vi "Read_Joint_States.vi"(0 "error in":errorcluster, 2 "Units (deg)":enum16{"Radians", "Degrees"}(ring)=enum."Degrees", 3 "node":string) -> (1 "error out":errorcluster, 4 "Joint States":T1(array[cluster]))   [LabVIEW 2015]
doc: "Read all the current joint states (names, positions, velocity, and efforts)"
uses:
  ROS/Code/Console/Servers/ServerSubs/TopicDef.ctl
  ROS/Code/SubVIs/_ROSDirection.ctl
panel:
  out "Reply":string
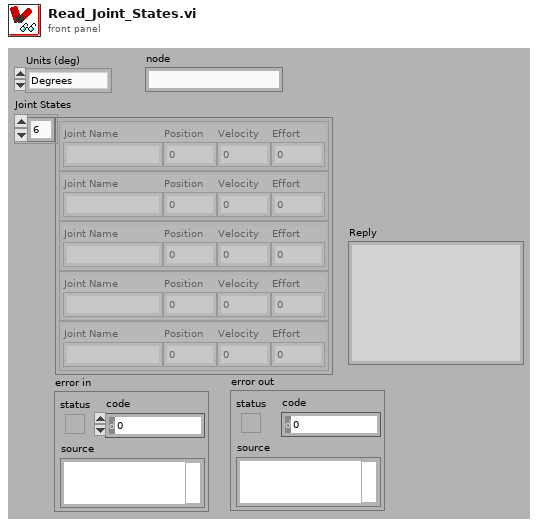
[diagram p1: front panel]
types:
  T1 = cluster{"Joint Name":string, "Position":dbl, "Velocity":dbl, "Effort":dbl}[]
  T2 = typedef "TopicDef.ctl" = cluster{"Topic":string, "Type":string, "Action":T3, "Update (ms)":u16, "queue size":u16}
  T3 = typedef "_ROSDirection.ctl" = enum16{"Node", "Publisher", "Subscriber", "ServiceClient", "ServiceProvider"}
  T4 = typedef "_ROSControl.ctl" = cluster{"topic port":u16, "Node":string, "topic":string, "type":string, "node port":u16, "error ":errorcluster, "Direction":T3, "Update (ms)":u16, "FIFO size":u16}
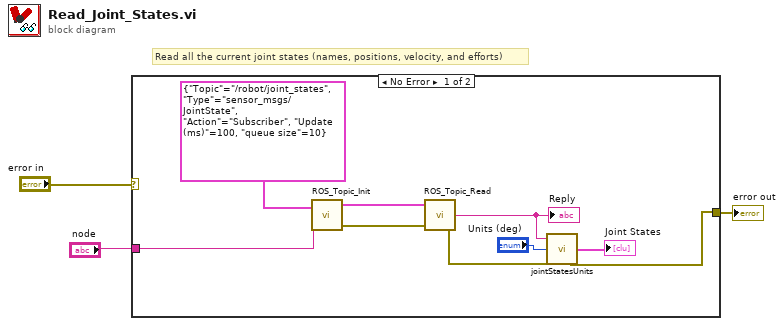
[diagram p0: block diagram]
diagram:
  # "Read all the current joint states (names, positions, velocity, and efforts)"
  n1 = case shown="No Error" "error in" {
    selector: "error in" -> [_ w13]
    tunnel: [w4 w13] -> w3
    tunnel: "node" -> [w7 _]
    frame No Error {
      n2 = call "ROS_Topic_Init.vi"("Definitions"=T2 {"Topic"="/robot/joint_states", "Type"="sensor_msgs/JointState", "Action"=enum."Subscriber", "Update (ms)"=100, "queue size"=10}, "node"=w7) -> ("ROS out"=w12:T4, "error out"=w6:errorcluster)  [unwired: 1 in]
      n3 = call "ROS_Topic_Read.vi"("error in (no error)"=w6, "ROS in"=w12) -> ("error out"=w5:errorcluster, "Reply"=w9:string)  [unwired: 1 in, 1 out]
      "Reply" <- w9
      n4 = call "jointStatesUnits.vi"("error in"=w5, "Units (deg)"="Units (deg)", "msg in"=w9) -> ("error out"=w4:errorcluster, "Joint States"=→"Joint States":T1)  [unwired: 1 out]
    }
    frame Error {
    }
  }
  "error out" <- w3
